vi "SetPinNumbering.vi"(5 "Pin Numbering":T1, 6 "error in":errorcluster) -> (0 "error out":errorcluster)   [LabVIEW 2014, in "GPIO.lvlib"]
doc: "This VI specifies which IO pin numbering system is to be used. BCM numbers refer to channel numbers on the Broadcom SOC. Board numbers refer to the pin numbers of the P1 header. If this VI is not called the default is BCM."
uses:
  GPIO.lvlib
  controls/PinNumbering.ctl
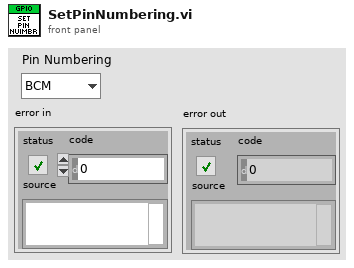
[diagram p1: front panel]
types:
  T1 = typedef "GPIO.lvlib/PinNumbering.ctl" = enum16{"BCM", "Board"}
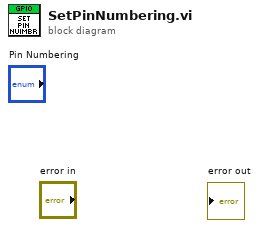
[diagram p0: block diagram]
diagram:
